vi "Create.vi"(10 "Path Statuses":T1[](array[typedef])) -> (3 "Git Path Status Value out":refnum<class "Git Path Status Value.lvclass">)   [LabVIEW 2020, in "VolatusGUI.lvlib" / "Git Path Status Value.lvclass"]
uses:
  Git Path Status Value.lvclass
  Git Path Status Value.lvclass/Git Path Status Value.ctl
  Git Updater Module/Status.ctl
  Git Updater Module/Git Updater Module.lvclass
  Git Updater Module/Path Status.ctl
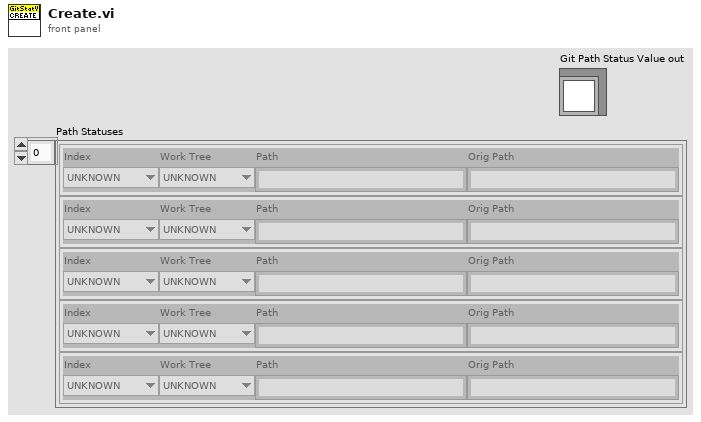
[diagram p1: front panel]
types:
  T1 = typedef "VolatusGUI.lvlib/Git Updater Module.lvclass/Path Status.ctl" = cluster{"Index":T2, "Work Tree":T2, "Path":string, "Orig Path":string}
  T2 = typedef "VolatusGUI.lvlib/Git Updater Module.lvclass/Status.ctl" = enum16{"UNKNOWN", "Unmodified", "Modified", "Added", "Deleted", "Renamed", "Unmerged", "Untracked", "Ignored"}
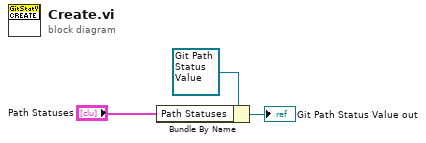
[diagram p0: block diagram]
diagram:
  n1 = Bundle By Name(cluster=refnum<class "Git Path Status Value.lvclass"> refnum ("Git Path Status Value in"), "Path Statuses"="Path Statuses") -> (→"Git Path Status Value out":refnum<class "Git Path Status Value.lvclass">)
